vi "array_average.vi"() -> ()   [LabVIEW 2025]
panel:
  out "Array Average":dbl
  in  "Array":dbl[](array[numeric])
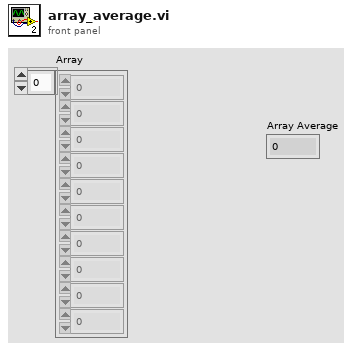
[diagram p1: front panel]
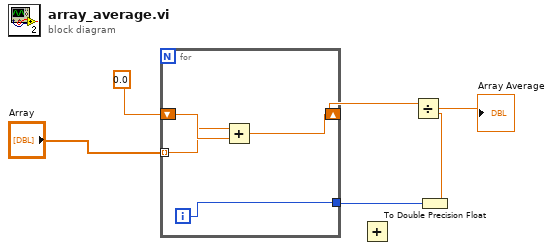
[diagram p0: block diagram]
diagram:
  n1 = for {
    tunnel: "Array" -> [w8] mode=indexing
    shift-right: [w10] -> w4
    shift-left: 0.0 -> [w9]
    tunnel: [w7] -> w2
    i -> [w7]
    n2 = Add(x=w8, y=w9) -> (x+y=w10:dbl)
  }
  n3 = Add() -> ()  [unwired: 2 in, 1 out]
  n4 = To Double Precision Float(number=w2) -> (double precision float=w3:dbl)
  n5 = Divide(x=w4, y=w3) -> (x/y=→"Array Average":dbl)
